vi "Ensure Visible.vi"(7 "#Layers":i32, 8 "error in (no error)":errorcluster, 11 "FakedArray in":refnum<class "FakedArray.lvclass">) -> (0 "error out":errorcluster, 3 "FakedArray out":refnum<class "FakedArray.lvclass">)   [LabVIEW 2020, in "FakedArray.lvclass"]
uses:
  FakedArray.lvclass
  FakedArray.lvclass/FakedArray.ctl
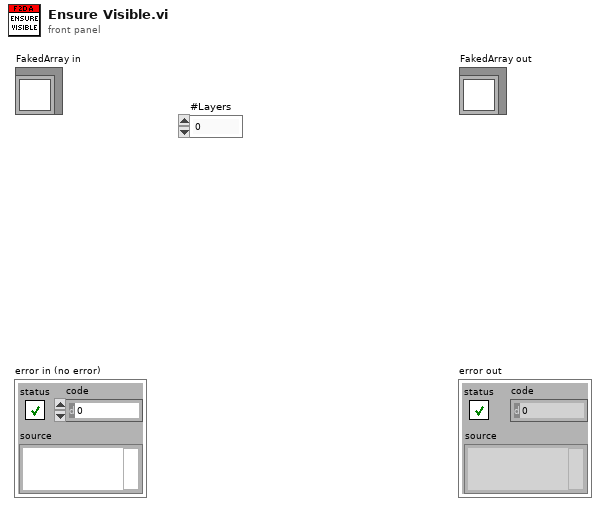
[diagram p1: front panel]
types:
  T1 = typedef "ToMoreSpecific_Faked2DArray.ctl" = enum16{"Framework Templates", "Layer List"}
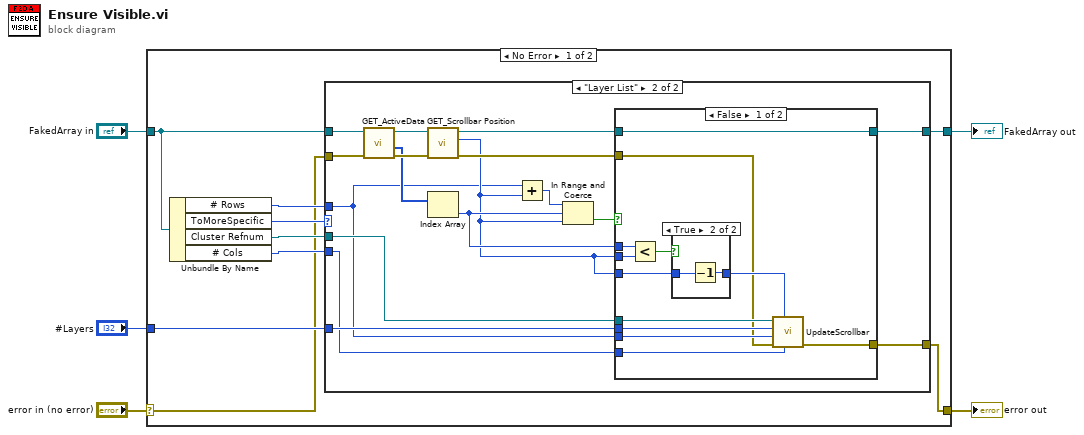
[diagram p0: block diagram]
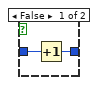
[diagram p3: hidden frame]
diagram:
  n1 = case shown="No Error" "error in (no error)" {
    selector: "error in (no error)" -> [w7 w53]
    tunnel: [w6 w53] -> w4
    tunnel: [w14 w52] -> w2
    tunnel: "FakedArray in" -> [w13 w52]
    tunnel: "#Layers" -> [w9 _]
    frame No Error {
      n2 = Unbundle By Name(w13) -> ("# Rows"=w11:i32, "ToMoreSpecific"=w12:T1, "Cluster Refnum"=w10:refnum<vi>, "# Cols"=w8:i32)
      n3 = case shown="\"Layer List\"" w12 {
        tunnel: w7 -> [w15 w33]
        tunnel: [w16 w23] -> w14
        tunnel: w13 -> [w16 w30]
        tunnel: w11 -> [_ w19]
        tunnel: w10 -> [_ w21]
        tunnel: w9 -> [_ w20]
        tunnel: w8 -> [_ w18]
        tunnel: [w15 w17] -> w6
        frame "Framework Templates", Default {
        }
        frame "Layer List" {
          n4 = call-dynamic "GET_ActiveData.vi"("error in (no error)"=w33, "FakedArray in"=w30) -> ("error out"=w31:errorcluster, "Active Data []"=w29:i32[], "FakedArray out"=w32:refnum<class "FakedArray.lvclass">)  [unwired: 7 out]
          n5 = call-dynamic "GET_Scrollbar Position.vi"("error in (no error)"=w31, "FakedArray.lvclass in"=w32) -> ("error out"=w26:errorcluster, "Scrollbar Position"=w22:i32, "FakedArray.lvclass out"=w27:refnum<class "FakedArray.lvclass">)  [unwired: 7 out]
          n6 = Index Array(array=w29) -> (element=w24:i32)  [unwired: 1 in]
          n7 = Add(x=w19, y=w22) -> (x+y=w28:i32)
          n8 = In Range and Coerce(upper limit=w28, x=w24, lower limit=w22) -> (In Range?=w25:bool)  [unwired: 1 out]
          n9 = case shown="False" w25 {
            tunnel: w27 -> [w44 w51]
            tunnel: w26 -> [w35 w50]
            tunnel: w24 -> [w43 _]
            tunnel: w22 -> [w45 _]
            tunnel: [w44 w51] -> w23
            tunnel: w22 -> [w41 _]
            tunnel: w21 -> [w39 _]
            tunnel: w20 -> [w38 _]
            tunnel: w19 -> [w37 _]
            tunnel: w18 -> [w36 _]
            tunnel: [w34 w50] -> w17
            frame False {
              n10 = Less?(x=w43, y=w45) -> (x < y?=w42:bool)
              n11 = case shown="True" w42 {
                tunnel: w41 -> [w47 w49]
                tunnel: [w46 w48] -> w40
                frame False {
                  n12 = Increment(x=w47) -> (x+1=w46:i32)
                }
                frame True {
                  n13 = Decrement(x=w49) -> (x-1=w48:i32)
                }
              }
              n14 = call "UpdateScrollbar.vi"("# Cols"=w36, "Value Scrollbar"=w40, "error in"=w35, "#Rows"=w37, "# Elements"=w38, "Cluster Refnum"=w39) -> ("error out"=w34:errorcluster)  [unwired: 5 out]
            }
            frame True {
            }
          }
        }
      }
    }
    frame Error {
    }
  }
  "error out" <- w4
  "FakedArray out" <- w2
